vi "Create Image.vi"   [LabVIEW 2020, in "g_ar_toolkit.lvlib"]
uses:
  g_ar_toolkit.lvlib
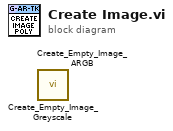
[diagram p0: block diagram]
diagram:
  n1 = call "Create_Empty_Image_Greyscale.vi"() -> ()  [unwired: 10 in, 2 out]
  n2 = call "Create_Empty_Image_ARGB.vi"() -> ()  [unwired: 10 in, 2 out]
